vi "ReadAllofMultiTiff_withtext.vi"(3 "error in":errorcluster, 5 "file path":path) -> (0 "error out":errorcluster, 1 "strings":string[](array[string]), 2 "16-bit pixmaps":i16[][][](array[numeric]))   [LabVIEW 2011]
uses:
  TiffModules/ReadTiffPage_I16_text.vi
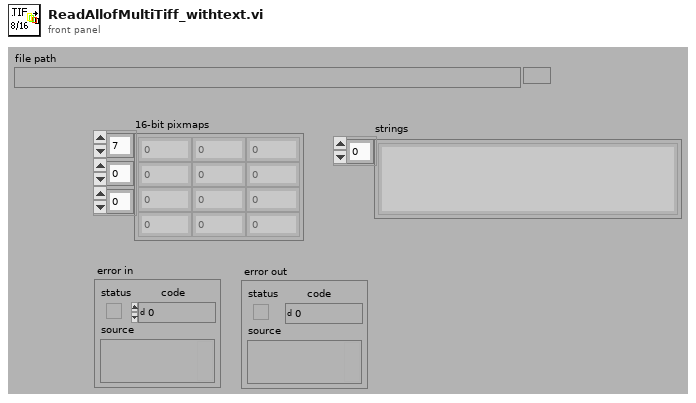
[diagram p1: front panel]
types:
  T1 = cluster{"Tiff refnum":refnum<file>, "BigTiff,Endian":u16}
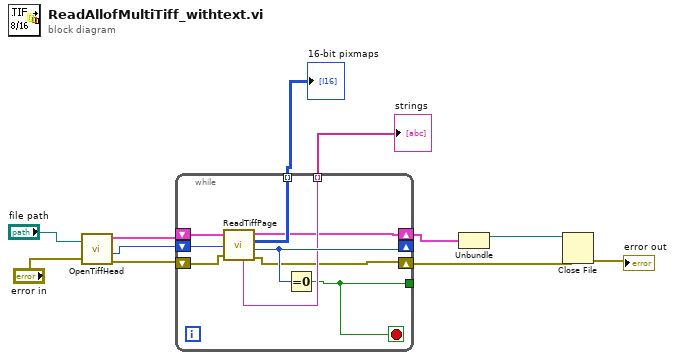
[diagram p0: block diagram]
diagram:
  n1 = call "OpenTiffHead.vi"("file path"="file path", "error in"="error in") -> ("TIFF file"=w8:T1, "first Diroffset"=w9:u64, "error out"=w7:errorcluster)  [unwired: 1 in]
  n2 = while {
    shift-right: [w17] -> _
    shift-left: w9 -> [w20]
    shift-right: [w13] -> w4
    shift-left: w8 -> [w19]
    shift-right: [w14] -> w3
    shift-left: w7 -> [w18]
    tunnel: [w12] -> _
    tunnel: [w16] -> w2 mode=indexing
    tunnel: [w15] -> w1 mode=indexing
    stop <- w12 stop-if-true
    n3 = call-poly "ReadTiffPage.vi"("TIFF file"=w19, "IFDoffset"=w20, "error in"=w18) -> ("TIFF file out"=w13:T1, "16-bit pixmap"=w16:i16[][], "string"=w15:string, "Next offset"=w17:i64, "error out"=w14:errorcluster)  [unwired: 3 in]
    n4 = Equal To 0?(x=w17) -> (x = 0?=w12:bool)
  }
  "strings" <- w1
  "16-bit pixmaps" <- w2
  n5 = Unbundle(w4) -> ("Tiff refnum"=w6:refnum<file>)  [unwired: 1 out]
  n6 = Close File(refnum=w6, error in=w3) -> (error out=→"error out":errorcluster)  [unwired: 1 out]
